vi "Create From Variant (Numeric).vi"(8 "error in (no error)":errorcluster, 10 "Variant":variant) -> (0 "error out":errorcluster, 3 "JSON Value out":refnum<class "JSON Value.lvclass">)   [LabVIEW 2016, in "JSFL Variant Support.lvlib"]
doc: "Creates a new JSON instance from the given Variant."
uses:
  JSFL Variant Support.lvlib
  JSON Value.lvclass
  New JSON Value/New JSON (Numeric).vi
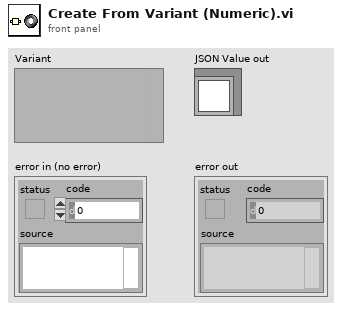
[diagram p1: front panel]
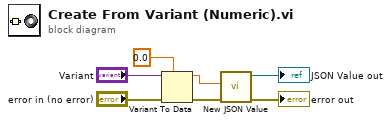
[diagram p0: block diagram]
diagram:
  n1 = Variant To Data(error in="error in (no error)", type=0.0, Variant="Variant") -> (data=w2:dbl, error out=w4:errorcluster)
  n2 = call-poly "New JSON Value.vi"("error in (no error)"=w4, "value"=w2) -> ("error out"=→"error out":errorcluster, "JSON Value out"=→"JSON Value out":refnum<class "JSON Value.lvclass">)  [unwired: 8 in]
